vi "ParaSet_2.vi"(11 "Controls":T1) -> (3 "String":string)   [LabVIEW 2014, in "Programing Logic.lvclass"]
uses:
  Programming Logic/Programing Logic.lvclass
  Controls/ParaSet.ctl
  Controls/Control Library.lvlib
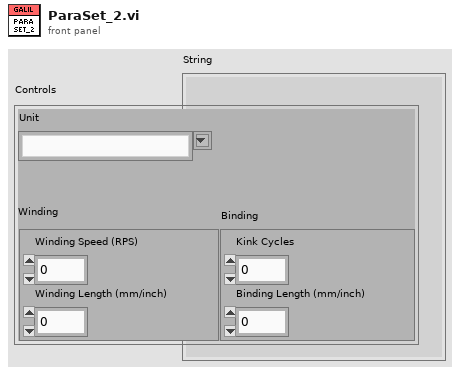
[diagram p1: front panel]
types:
  T1 = typedef "Control Library.lvlib/ParaSet.ctl" = cluster{"Unit":string, "Winding":cluster{"Winding Speed (RPS)":dbl, "Winding Length (mm/inch)":dbl}, "Binding":cluster{"Kink Cycles":dbl, "Binding Length (mm/inch)":dbl}}
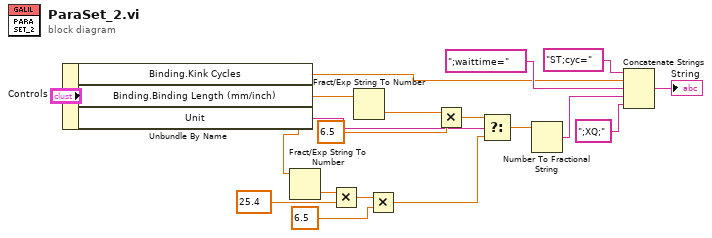
[diagram p0: block diagram]
diagram:
  n1 = Unbundle By Name("Controls") -> ("Binding.Kink Cycles"=w10:dbl, "Binding.Binding Length (mm/inch)"=w6:dbl, "Unit"=w7:string)
  n2 = Fract/Exp String To Number(string=w6) -> (number=w5:dbl)  [unwired: 3 in, 1 out]
  n3 = Multiply(x=w5, y=25.4) -> (x*y=w3:dbl)
  n4 = Fract/Exp String To Number(string=w6) -> (number=w14:dbl)  [unwired: 3 in, 1 out]
  n5 = Multiply(x=w3, y=6.5) -> (x*y=w1:dbl)
  n6 = Multiply(x=w14, y=6.5) -> (x*y=w9:dbl)
  n7 = Select(t=w9, s=w7, f=w1) -> (s? t:f=w8:dbl)
  n8 = Number To Fractional String(number=w8) -> (F-format string=w12:string)  [unwired: 3 in]
  n9 = Concatenate Strings("ST;cyc=" ("string"), w10, ";waittime=" ("string"), w12, ";XQ;" ("string")) -> (→"String":string)
